vi "Resolve Pin Map Path for Sequence.vi"(8 "error in":errorcluster, 10 "pin map path":path, 11 "sequence context in":refnum<k7>) -> (0 "error out":errorcluster, 2 "absolute pin map path":path, 3 "sequence context out":refnum<k7>)   [LabVIEW 2020, in "MeasurementLink Pin Map.lvlib"]
doc: "Attempts to resolve the <b>pin map path</b> to an absolute file path using standard TestStand search directories."
uses:
  MeasurementLink Pin Map.lvlib
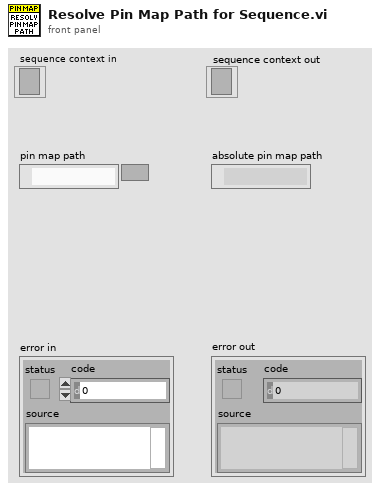
[diagram p1: front panel]
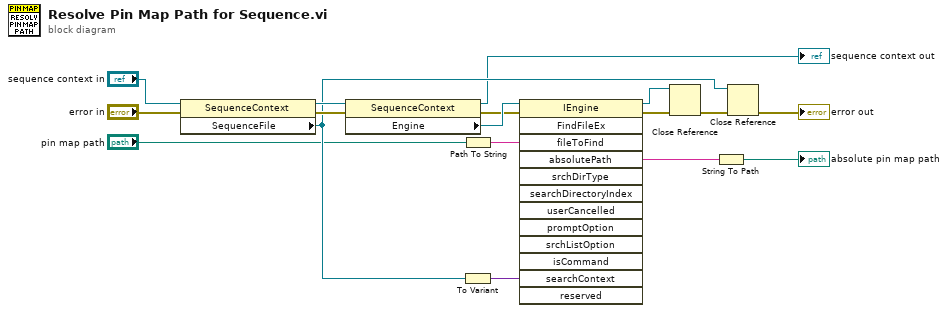
[diagram p0: block diagram]
diagram:
  n1 = property class="SequenceContext"(reference="sequence context in", error in="error in") -> (reference out=w10:refnum<k7>, error out=w12:errorcluster, "SequenceFile"=w7:refnum<k7>)
  n2 = property class="SequenceContext"(reference=w10, error in=w12) -> (reference out=→"sequence context out":refnum<k7>, error out=w16:errorcluster, "Engine"=w17:refnum<k7>)
  n3 = Path To String(path="pin map path") -> (string=w1:string)
  n4 = To Variant(anything=w7) -> (Variant=w6:variant)
  n5 = invoke class="IEngine" method="FindFileEx"(reference=w17, error in=w16, "fileToFind"=w1, "searchContext"=w6) -> (reference out=w15:refnum<k7>, error out=w14:errorcluster, "absolutePath"=w4:string)  [unwired: 9 in, 10 out]
  n6 = Close Reference(reference=w15, error in (no error)=w14) -> (error out=w9:errorcluster)
  n7 = String To Path(string=w4) -> (path=→"absolute pin map path":path)
  n8 = Close Reference(reference=w7, error in (no error)=w9) -> (error out=→"error out":errorcluster)
